vi "Write pattern.vi"(8 "error in (no error)":errorcluster, 10 "pattern":string, 11 "TreeDirectoryExt in":refnum<class "TreeDirectoryExt.lvclass">) -> (0 "error out":errorcluster, 3 "TreeDirectoryExt out":refnum<class "TreeDirectoryExt.lvclass">)   [LabVIEW 2026, in "TreeDirectoryExt.lvclass"]
uses:
  TreeDirectoryExt.lvclass
  TreeDirectoryExt.lvclass/TreeDirectoryExt.ctl
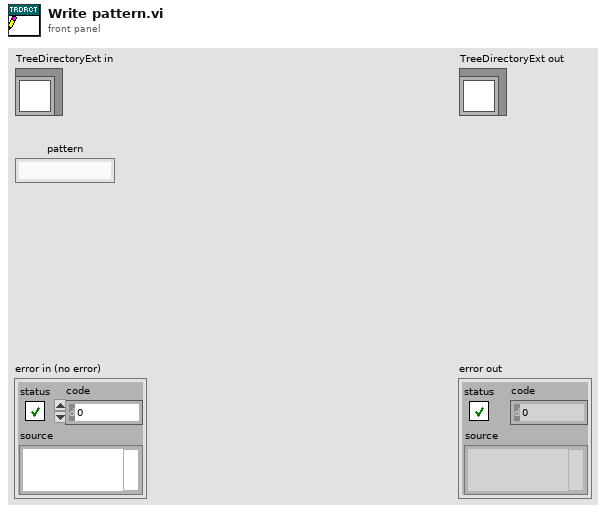
[diagram p1: front panel]
types:
  T1 = typedef "TreeDirectoryExt.lvclass/State Data.ctl" = cluster{"IconLibrary":variant, "pattern":string, "Clear Tree on Exit?":bool}
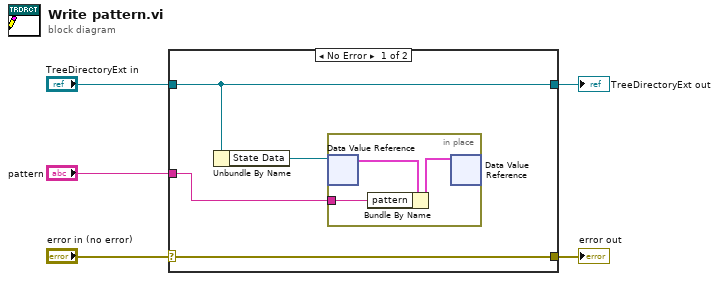
[diagram p0: block diagram]
diagram:
  n1 = case shown="No Error" "error in (no error)" {
    selector: "error in (no error)" -> [w9 w13]
    tunnel: [w9 w13] -> w4
    tunnel: [w6 w14] -> w2
    tunnel: "TreeDirectoryExt in" -> [w6 w14]
    tunnel: "pattern" -> [w7 _]
    frame No Error {
      n2 = Unbundle By Name(w6) -> ("State Data"=w8:refnum<data-value>)
      n3 = in-place {
        in-place-border: w7 -> [w10]
        n4 = in-place-dvr #1(w8) -> (w12:T1)  [unwired: 1 out]
        n5 = Bundle By Name(cluster=w12, "pattern"=w10) -> (w11:T1)
        n6 = in-place-dvr #1(w11) -> ()  [unwired: 2 out]
      }
    }
    frame Error {
    }
  }
  "error out" <- w4
  "TreeDirectoryExt out" <- w2
